vi "Analog Read PortTest.vi"() -> ()   [LabVIEW 2011]
uses:
  Private/Type Defs/Chipkit Configuration.ctl
  Private/Type Defs/Board Type.ctl
  Private/Type Defs/Analog Pin.ctl
  LabVIEW Interface for ChipKit.lvlib
panel:
  in  "Analog Pin":T1=enum."AI_3"
  out "Voltage":dbl
  in  "index":i32
  in  "ChipKit Configuration":T2
  out "Waveform Chart":dbl(graph)
  in  "Stop Button":bool
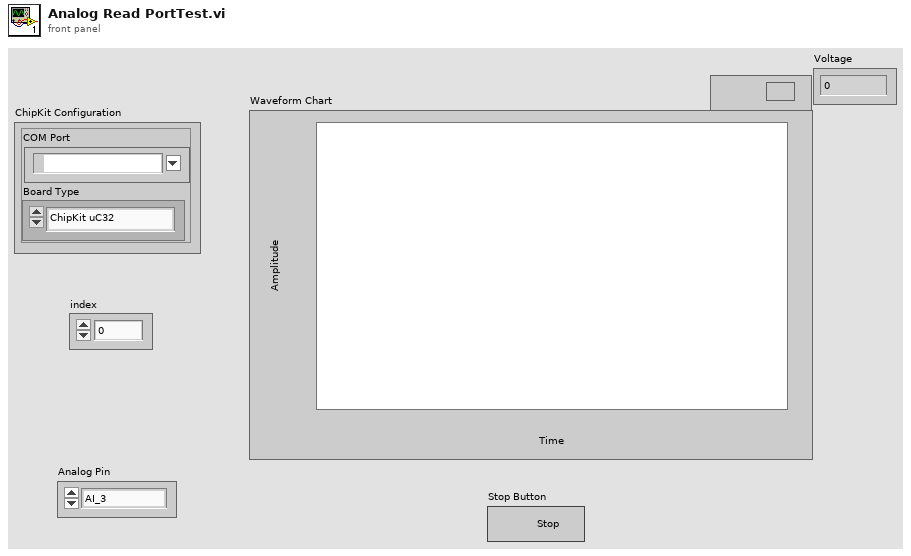
[diagram p1: front panel]
types:
  T1 = typedef "LabVIEW Interface for ChipKit.lvlib/Analog Pin.ctl" = enum16{"AI_0", "AI_1", "AI_2", "AI_3", "AI_4", "AI_5", "AI_6", "AI_7", "AI_8", "AI_9", "AI_10", "AI_11", "AI_12", "AI_13", "AI_14", "AI_15"}
  T2 = typedef "LabVIEW Interface for ChipKit.lvlib/Chipkit Configuration.ctl" = cluster{"COM Port":refnum<visa-resource-name>, "Board Type":T3}
  T3 = typedef "LabVIEW Interface for ChipKit.lvlib/Board Type.ctl" = enum16{"ChipKit uC32", "ChipKit Uno32", "ChipKit Max32"}
  T4 = typedef "LabVIEW Interface for ChipKit.lvlib/Chipkit Resource.ctl" = cluster{"COM Port":refnum<visa-resource-name>, "Board Type":T3, "Connection Type":T5, "Baud Rate (115200)":u32, "Bytes Per Packet (15)":u32, "DI Port Num Pins":i32, "DO Port Num Pins":i32}
  T5 = typedef "LabVIEW Interface for ChipKit.lvlib/Connection Type.ctl" = enum8{"USB / Serial", "XBEE", "BlueSmirf (Bluetooth)"}
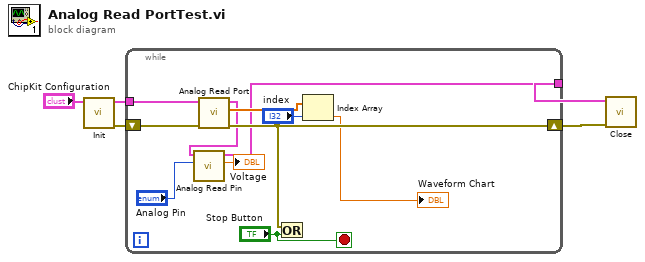
[diagram p0: block diagram]
diagram:
  n1 = call "Init.vi"("ChipKit Configuration"="ChipKit Configuration") -> ("Error Out"=w4:errorcluster, "ChipKit Configuration"=w5:T4)  [unwired: 9 in]
  n2 = while {
    tunnel: w5 -> [w16]
    shift-right: [w13] -> w2
    shift-left: w4 -> [w15]
    tunnel: [w8] -> w3
    stop <- "Stop Button" stop-if-true
    n3 = call "Analog Read Port.vi"("Error In"=w15, "ChipKit Resource"=w16) -> ("Error Out"=w13:errorcluster, "Analog Port"=w12:dbl[], "ChipKit Resource"=w9:T4)  [unwired: 7 in]
    n4 = call "Analog Read Pin.vi"("Analog Pin"="Analog Pin", "ChipKit Resource"=w9) -> ("Voltage"=→"Voltage":dbl, "ChipKit Resource"=w8:T4)  [unwired: 7 in, 1 out]
    n5 = Or(x=w13, y="Stop Button") -> ()  [unwired: 1 out]
    n6 = Index Array(array=w12, index="index") -> (element=→"Waveform Chart":dbl)
  }
  n7 = call "Close.vi"("Error In"=w2, "ChipKit Configuration"=w3) -> ()  [unwired: 9 in, 1 out]
